vi "Construct File Name.vi"(1 "Prefix":string, 7 "Binary Data":u8[](array[numeric])) -> (8 "File Name":string)   [LabVIEW 2017]
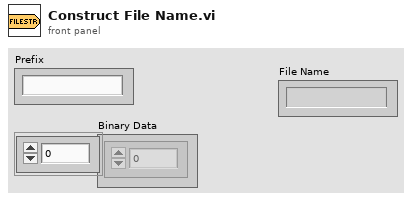
[diagram p1: front panel]
types:
  T1 = typedef "control_measurement_settings.ctl" = cluster{"# Pages":i32, "ODR":u8, "xlRange":u8, "gyroRange":u8, "id":u8, "Samplig Freq [Hz]":dbl, "xlRange in g":dbl, "gyroRange in dps":dbl}
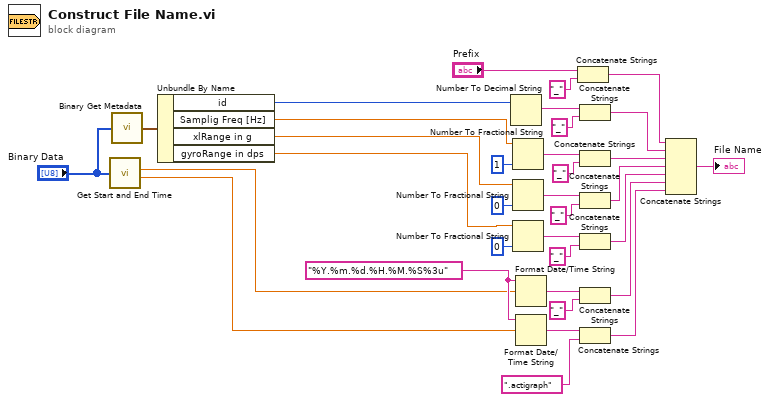
[diagram p0: block diagram]
diagram:
  w32 = "%Y.%m.%d.%H.%M.%S%3u" ("time format string (%c)")
  n1 = call "Get Start and End Time.vi"("Binary Data"="Binary Data") -> ("Start Time"=w1:dbl, "End Time"=w2:dbl)  [unwired: 8 in]
  n2 = call "Binary Get Metadata.vi"("Binary Data"="Binary Data") -> ("Meta"=w3:T1)  [unwired: 4 in]
  n3 = Unbundle By Name(w3) -> ("id"=w8:u8, "Samplig Freq [Hz]"=w7:dbl, "xlRange in g"=w6:dbl, "gyroRange in dps"=w5:dbl)
  n4 = Number To Decimal String(number=w8) -> (decimal integer string=w29:string)  [unwired: 1 in]
  n5 = Number To Fractional String(number=w7, precision (6)=i16 1) -> (F-format string=w27:string)  [unwired: 2 in]
  n6 = Number To Fractional String(number=w6, precision (6)=i16 0) -> (F-format string=w25:string)  [unwired: 2 in]
  n7 = Number To Fractional String(number=w5, precision (6)=i16 0) -> (F-format string=w23:string)  [unwired: 2 in]
  n8 = Format Date/Time String(time format string (%c)=w32, seconds (now)=w1) -> (date/time string=w20:string)  [unwired: 1 in]
  n9 = Format Date/Time String(time format string (%c)=w32, seconds (now)=w2) -> (date/time string=w31:string)  [unwired: 1 in]
  n10 = Concatenate Strings("Prefix", "_") -> (w9:string)
  n11 = Concatenate Strings(w29, "_") -> (w19:string)
  n12 = Concatenate Strings(w27, "_") -> (w18:string)
  n13 = Concatenate Strings(w25, "_") -> (w17:string)
  n14 = Concatenate Strings(w23, "_") -> (w16:string)
  n15 = Concatenate Strings(w20, "_") -> (w15:string)
  n16 = Concatenate Strings(w31, ".actigraph") -> (w14:string)
  n17 = Concatenate Strings(w9, w19, w18, w17, w16, w15, w14) -> (→"File Name":string)
